vi "read formatted default value.vi"(10 "# of Digits":u8=5, 11 "channel":refnum<class "TBM channel.lvclass">) -> (2 "Formatted Default":string, 3 "channel out":refnum<class "TBM channel.lvclass">)   [LabVIEW 2013, in "control module editor.lvclass"]
uses:
  control module editor.lvclass
  <vilib>/NI/Tag Bus Module Framework/channel/TBM channel.lvclass
  <vilib>/NI/Tag Bus/tag/tag descriptor.lvclass/tag descriptor.ctl
  <vilib>/NI/Tag Bus/tag/tag descriptor.lvclass
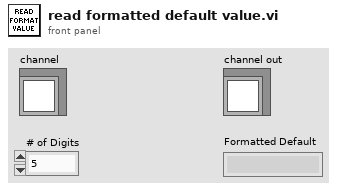
[diagram p1: front panel]
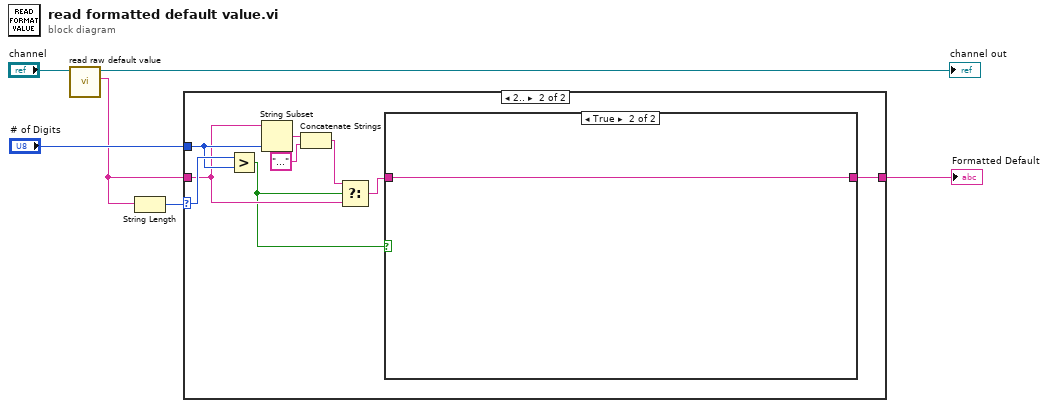
[diagram p0: block diagram]
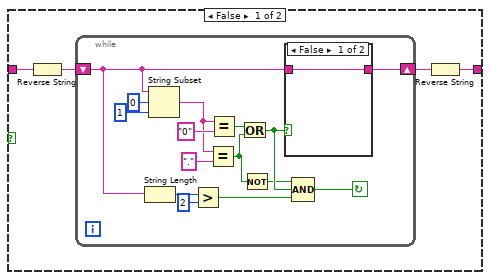
[diagram p3: hidden frame]
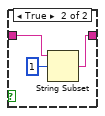
[diagram p4: hidden frame]
diagram:
  n1 = call <vilib>:"read raw default value.vi"("system tag in"="channel") -> ("raw default"=w3:string, "system tag out"=→"channel out":refnum<class "TBM channel.lvclass">)  [unwired: 8 in, 1 out]
  n2 = String Length(string=w3) -> (length=w5:i32)
  n3 = case shown="2.." w5 {
    selector: w5 -> [_ w12]
    tunnel: [w7 w16] -> w1
    tunnel: w3 -> [w7 w10]
    tunnel: "# of Digits" -> [_ w11]
    frame Default {
    }
    frame 2.. {
      n4 = Greater?(x=w12, y=w11) -> (0:w8:bool)
      n5 = String Subset(string=w10, length (rest)=w11) -> (substring=w14:string)  [unwired: 1 in]
      n6 = Concatenate Strings(w14, "..." ("string")) -> (w13:string)
      n7 = Select(t=w13, s=w8, f=w10) -> (s? t:f=w9:string)
      n8 = case shown="True" w8 {
        tunnel: [w18 w40] -> w16
        tunnel: w9 -> [w17 w40]
        frame False {
          n9 = Reverse String(1:w17) -> (0:w20:string)
          n10 = while {
            shift-right: [w29] -> w19
            shift-left: w20 -> [w28]
            stop <- w24 continue-if-true
            n11 = String Length(string=w28) -> (length=w27:i32)
            n12 = String Subset(string=w28, offset (0)=0, length (rest)=1 ("length (rest)")) -> (substring=w32:string)
            n13 = Greater?(x=w27, y=2) -> (0:w25:bool)
            n14 = Equal?(x=w32, y=".") -> (x = y?=w23:bool)
            n15 = Equal?(x=w32, y="0") -> (x = y?=w30:bool)
            n16 = Or(x=w30, y=w23) -> (x .or. y?=w22:bool)
            n17 = Not(x=w23) -> (.not. x?=w21:bool)
            n18 = case shown="False" w22 {
              tunnel: w28 -> [w36 w39]
              tunnel: [w36 w37] -> w29
              frame False {
              }
              frame True {
                n19 = String Subset(string=w39, offset (0)=1) -> (substring=w37:string)  [unwired: 1 in]
              }
            }
            n20 = Compound Arithmetic op=AND(w21, w22, w25) -> (w24:bool)
          }
          n21 = Reverse String(1:w19) -> (0:w18:string)
        }
        frame True {
        }
      }
    }
  }
  "Formatted Default" <- w1
